vi "GE 5565PIORC.Bit Manipulation.Get Bits (U16).vi"(8 "bit count (1)":i32=1, 9 "bit index":i32, 11 "packed value in":u16 format="%016x") -> (2 "bits":u16 format="%016x", 3 "packed value out":u16 format="%016x")   [LabVIEW 2020, in "GE 5565PIORC.lvclass"]
doc: "This VI extracts a subset of bits of length <B>bit count</B> from <B>packed value</B> starting at <B>bit index</B>."
uses:
  GE 5565PIORC.lvclass
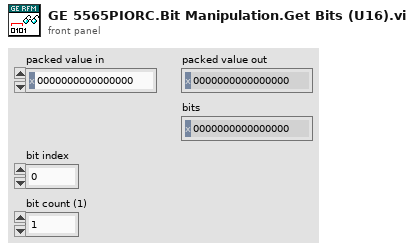
[diagram p1: front panel]
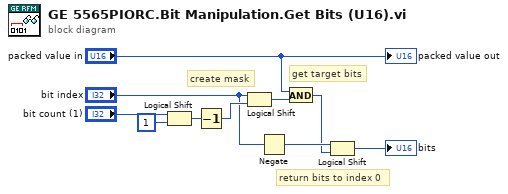
[diagram p0: block diagram]
diagram:
  # "return bits to index 0"
  # "create mask"
  # "get target bits"
  n1 = Logical Shift(y="bit count (1)", x=u16 1) -> (x << y=w9:u16)
  n2 = Decrement(x=w9) -> (x-1=w8:u16)
  n3 = Logical Shift(y="bit index", x=w8) -> (x << y=w6:u16)
  n4 = Negate(x="bit index") -> (-x=w3:i32)
  n5 = And(x="packed value in", y=w6) -> (x .and. y?=w2:u16)
  n6 = Logical Shift(y=w3, x=w2) -> (x << y=→"bits":u16)
  "packed value out" <- "packed value in"
